vi "Memory.Pointer.Error Handling.Out of Range.vi"(5 "parameter":T1, 7 "source vi name":string, 8 "error in (no error)":errorcluster, 10 "value":u64 format="%d bytes", 11 "Pointer in":refnum<class "Memory.Pointer.Void.lvclass">) -> (0 "error out":errorcluster, 3 "Pointer out":refnum<class "Memory.Pointer.Void.lvclass">)   [LabVIEW 2016, in "LabVIEW Memory Manager.lvlib" / "Memory.Pointer.Void.lvclass"]
uses:
  Memory.Pointer.Void.lvclass
  Typedefs/Memory.Pointer.Parameters.ctl
  Typedefs/Memory.Pointer.Error Codes.ctl
  RT Errors/VIs/Deterministic Errors.New Error Cluster (256B).vi
  RT Errors/VIs/Deterministic Errors.Write String to Source.vi
  RT Errors/Deterministic Errors.lvlib
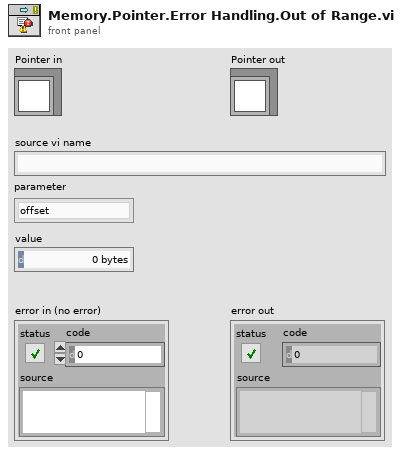
[diagram p1: front panel]
types:
  T1 = typedef "LabVIEW Memory Manager.lvlib/Memory.Pointer.Void.lvclass/Memory.Pointer.Parameters.ctl" = enum16{"offset", "length", "size", "subset"}
  T2 = typedef "LabVIEW Memory Manager.lvlib/Memory.Pointer.Void.lvclass/Memory.Pointer.Error Codes.ctl" = enum16{"Out of range"}
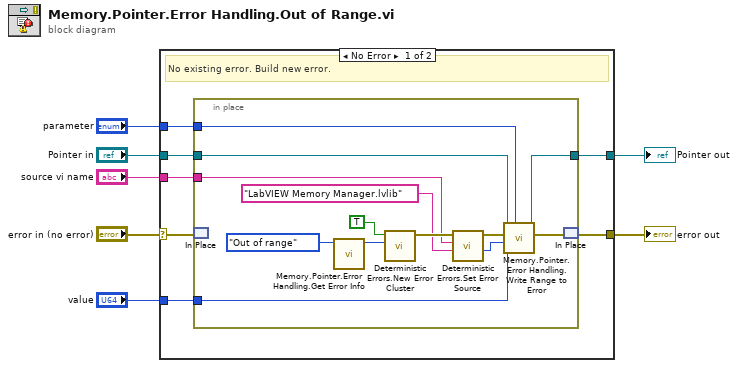
[diagram p0: block diagram]
diagram:
  n1 = case shown="No Error" "error in (no error)" {
    selector: "error in (no error)" -> [w13 w29]
    tunnel: [w14 w29] -> w4
    tunnel: "value" -> [w11 _]
    tunnel: "source vi name" -> [w12 _]
    tunnel: "parameter" -> [w10 _]
    tunnel: "Pointer in" -> [w9 w28]
    tunnel: [w8 w28] -> w1
    frame No Error {
      # "No existing error. Build new error."
      n2 = in-place {
        in-place-border: w12 -> [w24]
        in-place-border: w11 -> [w18]
        in-place-border: w10 -> [w15]
        in-place-border: w9 -> [w19]
        in-place-border: [w17] -> w8
        n3 = in-place-match #1(w13) -> ()  [unwired: 1 out]
        n4 = call "Memory.Pointer.Error Handling.Get Error Info.vi"("error"=Memory.Pointer.Error_Codes."Out of range" ("error code")) -> ("code"=w25:i32)  [unwired: 9 in, 1 out]
        n5 = call-poly "Deterministic Errors.New Error Cluster.vi"("code (0)"=w25, "status (F)"=TRUE) -> ("error out"=w27:errorcluster)  [unwired: 9 in]
        n6 = call "Deterministic Errors.Set Error Source.vi"("library name (\"\")"="LabVIEW Memory Manager.lvlib", "vi name"=w24, "error in"=w27) -> ("new offset"=w20:i32, "error out"=w21:errorcluster)  [unwired: 7 in]
        n7 = call "Memory.Pointer.Error Handling.Write Range to Error.vi"("parameter"=w15, "value"=w18, "offset"=w20, "error in"=w21, "Pointer in"=w19) -> ("error out"=w16:errorcluster, "Pointer out"=w17:refnum<class "Memory.Pointer.Void.lvclass">)  [unwired: 4 in, 1 out]
        n8 = in-place-match #1(w16) -> (w14:errorcluster)
      }
    }
    frame Error {
      # "Incoming error. Pass through."
    }
  }
  "error out" <- w4
  "Pointer out" <- w1
